vi "Write Group Index.vi"(8 "error in (no error)":errorcluster, 10 "Group Index":i32, 11 "Blackboard_Boolean in":refnum<class "Blackboard_Boolean.lvclass">) -> (0 "error out":errorcluster, 3 "Blackboard_Boolean out":refnum<class "Blackboard_Boolean.lvclass">)   [LabVIEW 2021, in "Blackboard_Boolean.lvclass"]
uses:
  Blackboard_Boolean.lvclass
  Blackboard_Boolean.lvclass/Blackboard_Boolean.ctl
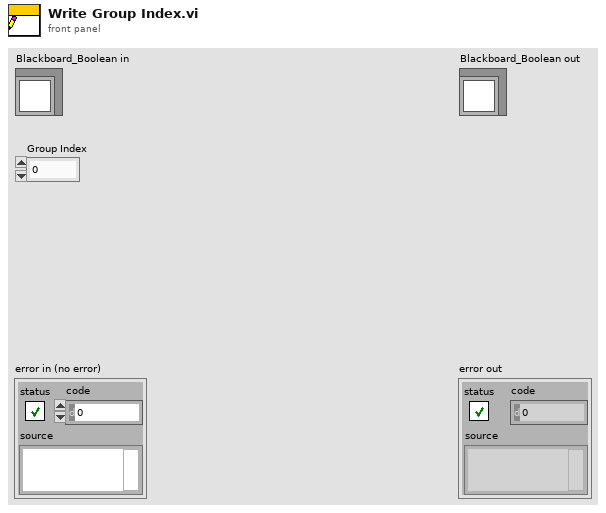
[diagram p1: front panel]
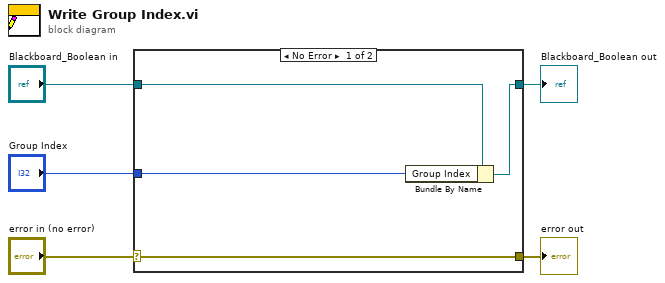
[diagram p0: block diagram]
diagram:
  n1 = case shown="No Error" "error in (no error)" {
    selector: "error in (no error)" -> [w9 w10]
    tunnel: [w9 w10] -> w4
    tunnel: [w7 w11] -> w2
    tunnel: "Blackboard_Boolean in" -> [w8 w11]
    tunnel: "Group Index" -> [w6 _]
    frame No Error {
      n2 = Bundle By Name(cluster=w8, "Group Index"=w6) -> (w7:refnum<class "Blackboard_Boolean.lvclass">)
    }
    frame Error {
    }
  }
  "error out" <- w4
  "Blackboard_Boolean out" <- w2
